vi "UltraScanning.vi"() -> ()   [LabVIEW 2014]
uses:
  <vilib>/userdefined/High Color/nirio_resource_hc.ctl
  <vilib>/Instr/_visa.llb/VISA Configure Serial Port (Instr).vi
  <vilib>/FPGAPlugInAG/PCIe-7851R/niLvFpga_Open_PCIe-7851R.vi
  <vilib>/rvi/interface/common/dynamic/niFpgaDynamicAddResources.vi
  <vilib>/Utility/error.llb/Error Cluster From Error Code.vi
  <vilib>/rvi/errors/niLvFpgaAdjustHostInterfaceError.vi
  <vilib>/FPGAPlugInAG/Dynamic/niLvFpga_Close_Dynamic.vi
  <vilib>/rvi/interface/nirviOpenFPGA/nirviOpenFPGA.xnode
  FPGA Bitfiles/FastHoppingModel_FPGATarget_StepApproach_dPgqUSt0PIw.lvbitx
  <vilib>/rvi/interface/nirviReadWriteControl/nirviReadWriteControl.xnode
  <vilib>/rvi/interface/nirviMethod/nirviMethod.xnode
  <vilib>/rvi/interface/nirviCloseFPGA/nirviCloseFPGA.xnode
  NiFpgaLv.dll
  <vilib>/rvi/interface/Simulation/niFpgaSimulationCallBeginRW.vi
  <vilib>/FPGAPlugInAG/Dynamic/niLvFpga_ReadFifo_Dynamic.vi
  <vilib>/rvi/errors/niLvFpgaMergeErrorWithErrorCode.vi
  CloseScanning.dll
  DeepScanning.dll
panel:
  out "Before":i16[][](array[numeric])
  out "After":u32[][](array[numeric])
  out "XNum?":i32
  out "YNum?":i32
  in  "SeveralSampleMeasure?":bool
  out "Intensity Graph":i32[][](graph)
  in  "Precise Scan Stop":bool
  out "RoughZPos um":dbl
  in  "steepWithdrawZIndex":i32
  in  "WithdrawZIndex":i32
  out "TimeDelta":u32
  in  "Prescan Stop":bool
  in  "PIZ":T1
  out "YPos um":dbl format="%#_13g"
  out "XPos um":dbl
  in  "InitOffset":i32
  in  "ApproachRate us":i32
  in  "Threshold %":dbl
  in  "YNum":i32
  in  "XNum":i32
  in  "XInitPos um":dbl
  in  "YInitPos um":dbl
  in  "YStepLen um":dbl
  in  "XStepLen um":dbl
  out "ERRIn?":string
  in  "RoughXYZ":refnum<visa-resource-name>
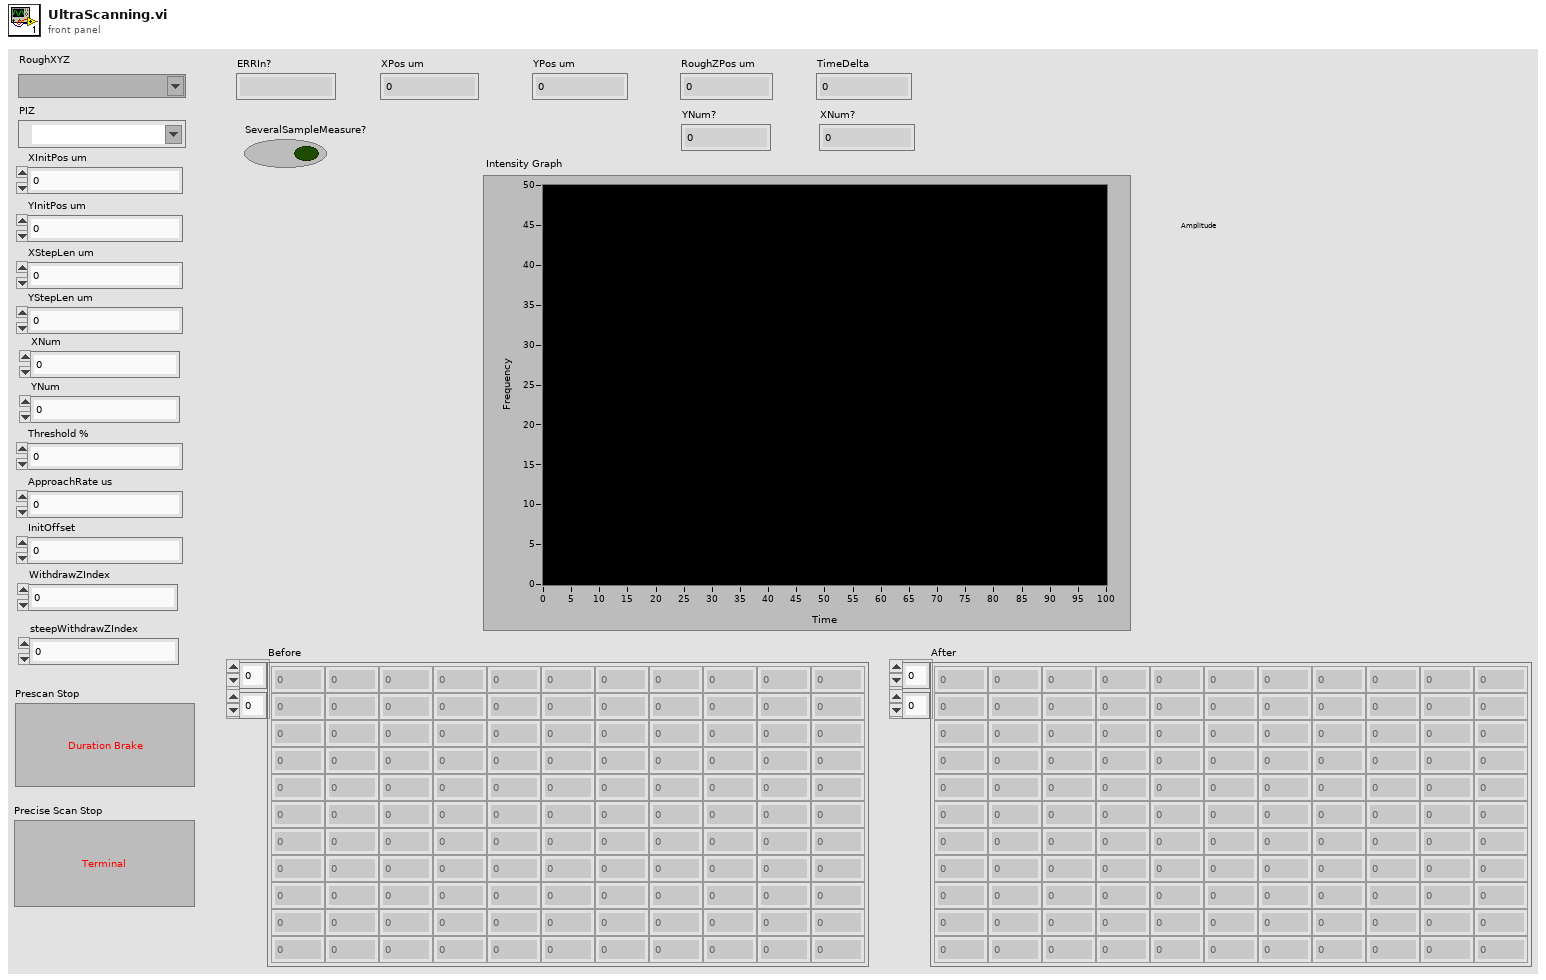
[diagram p1: front panel]
types:
  T1 = typedef "nirio_resource_hc.ctl" = tag
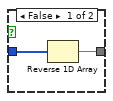
[diagram p2: hidden frame]
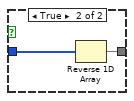
[diagram p5: hidden frame]
diagram:
  n1 = flat-sequence {
    tunnel: [w120] -> w98
    tunnel: [w119] -> w97
    tunnel: w98 -> [w148]
    tunnel: w97 -> [w147]
    tunnel: [w130] -> w96
    tunnel: [w129] -> w95
    tunnel: w96 -> [w150]
    tunnel: w95 -> [w149]
    tunnel: [w150] -> w94
    tunnel: [w149] -> w93
    tunnel: w94 -> [w177]
    tunnel: w93 -> [w176]
    tunnel: [w156] -> w92
    tunnel: [w155] -> w91
    tunnel: w92 -> [w179]
    tunnel: w91 -> [w178]
    tunnel: [w179] -> w90
    tunnel: [w178] -> w89
    tunnel: w90 -> [w189]
    tunnel: w89 -> [w188]
    tunnel: [w186] -> w88
    tunnel: [w185] -> w87
    tunnel: [w184] -> w86
    tunnel: [w183] -> w85
    tunnel: [w182] -> w84
    tunnel: [w181] -> w42
    tunnel: w88 -> [w401]
    tunnel: w87 -> [w403]
    tunnel: w86 -> [w402]
    tunnel: w85 -> [w399]
    tunnel: w84 -> [w398]
    tunnel: [w399] -> w49
    tunnel: [w398] -> w47
    tunnel: [w401] -> w45
    tunnel: [w400] -> w43
    tunnel: w42 -> [w400]
    tunnel: [w399] -> w41
    tunnel: [w398] -> w40
    tunnel: w49 -> [w410]
    tunnel: [w408] -> w48
    tunnel: w47 -> [w409]
    tunnel: [w407] -> w46
    tunnel: w45 -> [w412]
    tunnel: [w412] -> w44
    tunnel: w43 -> [w411]
    tunnel: w41 -> [w408]
    tunnel: w40 -> [w407]
    tunnel: w48 -> [w449]
    tunnel: w46 -> [w448]
    tunnel: w44 -> [w447]
    tunnel: [w449] -> w81
    tunnel: [w448] -> w79
    tunnel: [w436] -> w77
    tunnel: [w434] -> w74
    tunnel: [w438] -> w73
    tunnel: [w437] -> w72
    tunnel: [w439] -> w66
    tunnel: [w443] -> w64
    tunnel: [w442] -> w62
    tunnel: [w432] -> w60
    tunnel: [w435] -> w8
    tunnel: [w433] -> w7
    tunnel: [w431] -> w1
    tunnel: w81 -> [w465]
    tunnel: [w465] -> w80
    tunnel: w79 -> [w464]
    tunnel: [w464] -> w78
    tunnel: w77 -> [w463]
    tunnel: [w463] -> w76
    tunnel: [w462] -> w75
    tunnel: w74 -> [w457]
    tunnel: w73 -> [w459]
    tunnel: w72 -> [w458]
    tunnel: [w459] -> w71
    tunnel: [w458] -> w70
    tunnel: [w457] -> w69
    tunnel: [w456] -> w68
    tunnel: [w455] -> w67
    tunnel: w66 -> [w455]
    tunnel: [w454] -> w65
    tunnel: w64 -> [w453]
    tunnel: [w453] -> w63
    tunnel: w62 -> [w452]
    tunnel: [w452] -> w61
    tunnel: w60 -> [w451]
    tunnel: [w451] -> w59
    tunnel: [w450] -> w57
    tunnel: w8 -> [w462]
    tunnel: w7 -> [w456]
    tunnel: w1 -> [w450]
    tunnel: w80 -> [w486]
    tunnel: w78 -> [w485]
    tunnel: w76 -> [w476]
    tunnel: w75 -> [w475]
    tunnel: [w486] -> w83
    tunnel: [w485] -> w82
    tunnel: w71 -> [w481]
    tunnel: w70 -> [w480]
    tunnel: w69 -> [w474]
    tunnel: w68 -> [w473]
    tunnel: w67 -> [w482]
    tunnel: w65 -> [w477]
    tunnel: w63 -> [w479]
    tunnel: w61 -> [w478]
    tunnel: w59 -> [w484]
    tunnel: [w484] -> w58
    tunnel: w57 -> [w483]
    tunnel: [w483] -> w56
    tunnel: [w469] -> w6
    tunnel: [w467] -> w5
    tunnel: [w466] -> w4
    tunnel: [w470] -> w3
    tunnel: [w468] -> w2
    tunnel: w83 -> [w504]
    tunnel: w82 -> [w503]
    tunnel: w58 -> [w492]
    tunnel: w56 -> [w491]
    tunnel: [w501] -> w55
    tunnel: [w500] -> w54
    tunnel: [w493] -> w38
    tunnel: [w492] -> w36
    tunnel: [w491] -> w33
    tunnel: [w490] -> w30
    tunnel: [w489] -> w27
    tunnel: [w488] -> w26
    tunnel: [w487] -> w21
    tunnel: w6 -> [w493]
    tunnel: w5 -> [w489]
    tunnel: w4 -> [w488]
    tunnel: w3 -> [w487]
    tunnel: w2 -> [w490]
    tunnel: w55 -> [w513]
    tunnel: w54 -> [w512]
    tunnel: [w513] -> w53
    tunnel: [w512] -> w52
    tunnel: [w511] -> w39
    tunnel: w38 -> [w511]
    tunnel: w36 -> [w510]
    tunnel: [w510] -> w34
    tunnel: w33 -> [w509]
    tunnel: [w509] -> w32
    tunnel: w30 -> [w508]
    tunnel: [w508] -> w29
    tunnel: w27 -> [w507]
    tunnel: w26 -> [w506]
    tunnel: [w507] -> w25
    tunnel: [w506] -> w23
    tunnel: w21 -> [w505]
    tunnel: [w505] -> w20
    tunnel: w53 -> [w548]
    tunnel: w52 -> [w547]
    tunnel: [w525] -> w51
    tunnel: [w524] -> w50
    tunnel: w39 -> [w521]
    tunnel: [w521] -> w37
    tunnel: [w520] -> w35
    tunnel: w34 -> [w520]
    tunnel: w32 -> [w519]
    tunnel: [w519] -> w31
    tunnel: w29 -> [w518]
    tunnel: [w518] -> w28
    tunnel: w25 -> [w517]
    tunnel: [w517] -> w24
    tunnel: w23 -> [w516]
    tunnel: [w516] -> w22
    tunnel: w20 -> [w515]
    tunnel: [w515] -> w19
    tunnel: w51 -> [w561]
    tunnel: w50 -> [w560]
    tunnel: w37 -> [w562]
    tunnel: w35 -> [w556]
    tunnel: w31 -> [w555]
    tunnel: w28 -> [w559]
    tunnel: w24 -> [w557]
    tunnel: w22 -> [w558]
    tunnel: w19 -> [w553]
    tunnel: [w552] -> w18
    tunnel: [w551] -> w16
    tunnel: [w550] -> w14
    tunnel: [w549] -> w12
    tunnel: w18 -> [w810]
    tunnel: [w810] -> w17
    tunnel: w16 -> [w809]
    tunnel: [w809] -> w15
    tunnel: w14 -> [w808]
    tunnel: [w808] -> w13
    tunnel: w12 -> [w807]
    tunnel: [w807] -> w11
    tunnel: w17 -> [_]
    tunnel: w15 -> [_]
    tunnel: w13 -> [w815]
    tunnel: w11 -> [w814]
    tunnel: [w812] -> w10
    tunnel: [w811] -> w9
    tunnel: w10 -> [w824]
    tunnel: w9 -> [w823]
    frame #0 {
      w106 = 0 ("x")
      n2 = Wait (ms)(milliseconds to wait=u32 1000) -> ()  [unwired: 1 out]
      n3 = local write "XNum"("XNum") -> ()
      n4 = local write "InitOffset"("InitOffset") -> ()
      n5 = local write "YNum"("YNum") -> ()
      n6 = local write "Threshold %"("Threshold %") -> ()
      n7 = local write "XInitPos um"("XInitPos um") -> ()
      n8 = local write "XStepLen um"("XStepLen um") -> ()
      n9 = local write "YInitPos um"("YInitPos um") -> ()
      n10 = local write "YStepLen um"("YStepLen um") -> ()
      n11 = local write "ApproachRate us"("ApproachRate us") -> ()
      n12 = Equal?(x=w106, y="steepWithdrawZIndex") -> (x = y?=w100:bool)
      n13 = Equal?(x=w106, y="WithdrawZIndex") -> (x = y?=w105:bool)
      n14 = call-poly "VISA Configure Serial Port"("VISA resource name"="RoughXYZ", "baud rate (9600)"=u32 115200) -> ("VISA resource name out"=w126:refnum<visa-resource-name>, "error out"=w125:errorcluster)  [unwired: 12 in]
      n15 = Select(t=400 ("x"), s=w105, f="WithdrawZIndex") -> (s? t:f=w103:i32)
      n16 = Select(t=1000 ("x"), s=w100, f="steepWithdrawZIndex") -> (s? t:f=w102:i32)
      n17 = local write "steepWithdrawZIndex"(w102) -> ()
      n18 = local write "WithdrawZIndex"(w103) -> ()
      n19 = VISA Write(VISA resource name=w126, write buffer="ERR?\n", error in (no error)=w125) -> (VISA resource name out=w123:refnum<visa-resource-name>, error out=w122:errorcluster)  [unwired: 1 out]
      n20 = VISA Read(VISA resource name=w123, byte count=u32 128, error in (no error)=w122) -> (VISA resource name out=w120:refnum<visa-resource-name>, read buffer=→"ERRIn?":string, error out=w119:errorcluster)  [unwired: 1 out]
    }
    frame #1 {
      w140 = "\n" ("string")
      n21 = local read "YInitPos um"() -> (w135:dbl)
      n22 = local read "XInitPos um"() -> (w138:dbl)
      n23 = Wait (ms)(milliseconds to wait=u32 100) -> ()  [unwired: 1 out]
      n24 = Number To Fractional String(number=w135, precision (6)=i16 10) -> (F-format string=w134:string)  [unwired: 2 in]
      n25 = Number To Fractional String(number=w138, precision (6)=i16 10) -> (F-format string=w133:string)  [unwired: 2 in]
      n26 = Concatenate Strings("MOV B " ("string"), w134, w140) -> (w131:string)
      n27 = Concatenate Strings("MOV A " ("string"), w133, w140) -> (w132:string)
      n28 = Concatenate Strings(w132, w131) -> (w142:string)
      n29 = VISA Write(VISA resource name=w148, write buffer="ONL 1 1 2 1 3 1\nSVO A 1\nSVO B 1\nSVO C 1\nMOV C 0\n", error in (no error)=w147) -> (VISA resource name out=w144:refnum<visa-resource-name>, error out=w143:errorcluster)  [unwired: 1 out]
      n30 = VISA Write(VISA resource name=w144, write buffer=w142, error in (no error)=w143) -> (VISA resource name out=w130:refnum<visa-resource-name>, error out=w129:errorcluster)  [unwired: 1 out]
    }
    frame #2 {
      n31 = Wait (ms)(milliseconds to wait=u32 100) -> ()  [unwired: 1 out]
    }
    frame #3 {
      w153 = 2 ("offset")
      w157 = u32 128 ("byte count")
      n32 = VISA Write(VISA resource name=w177, write buffer="POS? A\n", error in (no error)=w176) -> (VISA resource name out=w174:refnum<visa-resource-name>, error out=w173:errorcluster)  [unwired: 1 out]
      n33 = VISA Read(VISA resource name=w174, byte count=w157, error in (no error)=w173) -> (VISA resource name out=w172:refnum<visa-resource-name>, read buffer=w170:string, error out=w171:errorcluster)  [unwired: 1 out]
      n34 = Fract/Exp String To Number(string=w170, offset=2) -> (number=→"XPos um":dbl)  [unwired: 2 in, 1 out]
      n35 = VISA Write(VISA resource name=w172, write buffer="POS? B\n", error in (no error)=w171) -> (VISA resource name out=w167:refnum<visa-resource-name>, error out=w166:errorcluster)  [unwired: 1 out]
      n36 = VISA Read(VISA resource name=w167, byte count=w157, error in (no error)=w166) -> (VISA resource name out=w162:refnum<visa-resource-name>, read buffer=w164:string, error out=w161:errorcluster)  [unwired: 1 out]
      n37 = Fract/Exp String To Number(string=w164, offset=w153) -> (number=→"YPos um":dbl)  [unwired: 2 in, 1 out]
      n38 = VISA Write(VISA resource name=w162, write buffer="POS? C\n", error in (no error)=w161) -> (VISA resource name out=w159:refnum<visa-resource-name>, error out=w158:errorcluster)  [unwired: 1 out]
      n39 = VISA Read(VISA resource name=w159, byte count=w157, error in (no error)=w158) -> (VISA resource name out=w156:refnum<visa-resource-name>, read buffer=w154:string, error out=w155:errorcluster)  [unwired: 1 out]
      n40 = Fract/Exp String To Number(string=w154, offset=w153) -> (number=→"RoughZPos um":dbl)  [unwired: 2 in, 1 out]
    }
    frame #4 {
      n41 = Wait (ms)(milliseconds to wait=u32 100) -> ()  [unwired: 1 out]
    }
    frame #5 {
      n42 = local read "YNum"() -> (w190:i32)
      n43 = for {
        N: w190 -> [_]
        tunnel: w189 -> [w224]
        tunnel: w188 -> [w223]
        shift-right: [w211] -> _
        shift-left: 0 -> [w217]
        tunnel: [w197] -> w183
        tunnel: [w196] -> w182
        tunnel: [w195] -> w185 mode=indexing
        tunnel: [w194] -> w184 mode=indexing
        tunnel: [w193] -> w186 mode=indexing
        tunnel: [w192] -> w181
        i -> [w191]
        stop <- w192 stop-if-true
        n44 = flat-sequence {
          tunnel: w191 -> [w249]
          tunnel: [w243] -> w225
          tunnel: w224 -> [w242]
          tunnel: w223 -> [w241]
          tunnel: [w240] -> w222
          tunnel: [w239] -> w221
          tunnel: w191 -> [w232]
          tunnel: [w228] -> w218
          tunnel: w217 -> [w228]
          tunnel: [w227] -> w206
          tunnel: w191 -> [w226]
          tunnel: w225 -> [w251]
          tunnel: w222 -> [w254]
          tunnel: w221 -> [w253]
          tunnel: [w254] -> w220
          tunnel: [w253] -> w219
          tunnel: w218 -> [w252]
          tunnel: [w252] -> w216
          tunnel: [w251] -> w215
          tunnel: [w250] -> w207
          tunnel: w206 -> [w250]
          tunnel: w220 -> [w268]
          tunnel: w219 -> [w267]
          tunnel: w216 -> [w265]
          tunnel: w215 -> [w266]
          tunnel: [w263] -> w214
          tunnel: [w262] -> w212
          tunnel: [w261] -> w209
          tunnel: w207 -> [w260]
          tunnel: [w260] -> w204
          tunnel: [w259] -> w202
          tunnel: [w258] -> w200
          tunnel: [w257] -> w198
          tunnel: w214 -> [w375]
          tunnel: [w375] -> w213
          tunnel: w212 -> [w374]
          tunnel: [w374] -> w210
          tunnel: w209 -> [w373]
          tunnel: [w373] -> w208
          tunnel: [w372] -> w205
          tunnel: w204 -> [w372]
          tunnel: [w371] -> w203
          tunnel: w202 -> [w371]
          tunnel: [w370] -> w201
          tunnel: w200 -> [w370]
          tunnel: [w368] -> w199
          tunnel: w198 -> [w368]
          tunnel: w213 -> [w393]
          tunnel: [w392] -> w211
          tunnel: w210 -> [w392]
          tunnel: [w391] -> w192
          tunnel: w208 -> [w391]
          tunnel: w205 -> [w390]
          tunnel: w203 -> [w383]
          tunnel: w201 -> [w382]
          tunnel: w199 -> [w389]
          tunnel: [w388] -> w193
          tunnel: [w381] -> w197
          tunnel: [w380] -> w196
          tunnel: [w379] -> w195
          tunnel: [w376] -> w194
          frame #0 {
            n45 = local read "YStepLen um"() -> (w233:dbl)
            n46 = local read "YInitPos um"() -> (w231:dbl)
            n47 = Multiply(x=w232, y=w233) -> (x*y=w230:dbl)
            n48 = Add(x=w231, y=w230) -> (x+y=w229:dbl)
            n49 = Number To Fractional String(number=w229, precision (6)=i16 10) -> (F-format string=w234:string)  [unwired: 2 in]
            n50 = Quotient & Remainder(x=w249, y=2) -> (x-y*floor(x/y)=w247:i32)  [unwired: 1 out]
            n51 = Concatenate Strings("MOV B " ("string"), w234, "\n" ("string")) -> (w238:string)
            n52 = Equal?(x=w247, y=0) -> (x = y?=w227:bool)
            n53 = VISA Write(VISA resource name=w242, write buffer=w238, error in (no error)=w241) -> (VISA resource name out=w240:refnum<visa-resource-name>, error out=w239:errorcluster)  [unwired: 1 out]
            n54 = Select(t=1, s=w227, f=-1) -> (s? t:f=w243:i32)
            "YNum?" <- w226
          }
          frame #1 {
            n55 = Wait (ms)(milliseconds to wait=u32 5) -> ()  [unwired: 1 out]
          }
          frame #2 {
            n56 = local read "XNum"() -> (w264:i32)
            n57 = Tick Count (ms)() -> (millisecond timer value=w256:u32)
            n58 = for {
              N: w264 -> [_]
              tunnel: w268 -> [w305]
              tunnel: w267 -> [w304]
              tunnel: w266 -> [w303]
              tunnel: w265 -> [w275]
              tunnel: [w278] -> w259
              tunnel: [w277] -> w258
              tunnel: [w276] -> w263 mode=indexing
              tunnel: [w274] -> w262
              tunnel: [w273] -> w261
              tunnel: [w271] -> w257 mode=indexing
              shift-right: [w269] -> _
              shift-left: w256 -> [w270]
              i -> [w302]
              stop <- w273 stop-if-true
              n59 = local read "XStepLen um"() -> (w300:dbl)
              n60 = Multiply(x=w302, y=w303) -> (x*y=w301:i32)
              n61 = local read "XInitPos um"() -> (w298:dbl)
              n62 = Add(x=w275, y=w301) -> (x+y=w274:i32)
              n63 = Multiply(x=w300, y=w274) -> (x*y=w299:dbl)
              n64 = Add(x=w298, y=w299) -> (x+y=w297:dbl)
              n65 = flat-sequence {
                tunnel: w305 -> [w315]
                tunnel: w304 -> [w314]
                tunnel: w297 -> [w309]
                tunnel: [w307] -> w296
                tunnel: [w306] -> w295
                tunnel: w296 -> [w317]
                tunnel: w295 -> [w316]
                tunnel: [w317] -> w294
                tunnel: [w316] -> w293
                tunnel: w294 -> [w326]
                tunnel: w293 -> [w325]
                tunnel: [w328] -> w292
                tunnel: [w327] -> w291
                tunnel: [w326] -> w290
                tunnel: [w325] -> w289
                tunnel: w292 -> [w343]
                tunnel: w291 -> [w342]
                tunnel: w290 -> [w336]
                tunnel: w289 -> [w335]
                tunnel: [w337] -> w288
                tunnel: [w336] -> w285
                tunnel: [w335] -> w283
                tunnel: [w334] -> w281
                tunnel: [w333] -> w279
                tunnel: ["Prescan Stop"] -> w273
                tunnel: w288 -> [w348]
                tunnel: [w348] -> w287
                tunnel: [w347] -> w286
                tunnel: w285 -> [w347]
                tunnel: [w346] -> w284
                tunnel: w283 -> [w346]
                tunnel: [w345] -> w282
                tunnel: w281 -> [w345]
                tunnel: [w344] -> w280
                tunnel: w279 -> [w344]
                tunnel: w287 -> [w356]
                tunnel: w286 -> [w365]
                tunnel: w284 -> [w364]
                tunnel: w282 -> [w367]
                tunnel: w280 -> [w366]
                tunnel: [w360] -> w278
                tunnel: [w359] -> w277
                tunnel: [w355] -> w271
                tunnel: [w352] -> w276
                tunnel: [w351] -> w269
                frame #0 {
                  n66 = Number To Fractional String(number=w309, precision (6)=i16 10) -> (F-format string=w308:string)  [unwired: 2 in]
                  n67 = Concatenate Strings("MOV B " ("string"), w308, "\n" ("string")) -> (w311:string)
                  n68 = VISA Write(VISA resource name=w315, write buffer=w311, error in (no error)=w314) -> (VISA resource name out=w307:refnum<visa-resource-name>, error out=w306:errorcluster)  [unwired: 1 out]
                }
                frame #1 {
                  n69 = Wait (ms)(milliseconds to wait=u32 5) -> ()  [unwired: 1 out]
                }
                frame #2 {
                  n70 = local read "ApproachRate us"() -> (w322:i32)
                  n71 = local read "Threshold %"() -> (w324:dbl)
                  n72 = local read "InitOffset"() -> (w323:i32)
                  n73 = xnode "Open FPGA VI Reference"("resource name"="PIZ") -> ("FPGA VI Reference Out"=w330:refnum<k20>, "error out"=w329:errorcluster)  [unwired: 1 in]
                  n74 = xnode "Read/Write Control"("FPGA VI Reference In"=w330, "error in"=w329, "Percentage %"=w324, "Offset"=w323, "AppRate us"=w322, "BaseTime us"=500, "CurrSampleNum"=100, "SeveralSampleMeasure?"="SeveralSampleMeasure?") -> ("FPGA VI Reference Out"=w328:refnum<k20>, "error out"=w327:errorcluster)
                }
                frame #3 {
                  n75 = xnode "Read/Write Control"("FPGA VI Reference In"=w343, "error in"=w342, "stop"="Prescan Stop") -> ("FPGA VI Reference Out"=w341:refnum<k20>, "error out"=w340:errorcluster)
                  n76 = xnode "Invoke Method"("FPGA VI Reference In"=w341, "error in"=w340, "Number of Elements"=u32 1, "Timeout (ms)"=7000) -> ("FPGA VI Reference Out"=w334:refnum<k20>, "error out"=w333:errorcluster, "Data"=w337:i16[])  [unwired: 1 out]
                }
                frame #4 {
                  n77 = Wait (ms)(milliseconds to wait=u32 1) -> ()  [unwired: 1 out]
                }
                frame #5 {
                  n78 = xnode "Close FPGA VI Reference"("FPGA VI Reference In"=w367, "error in"=w366) -> ()  [unwired: 1 out]
                  n79 = Array Size(array=w356) -> (size(s)=w358:i32)
                  n80 = VISA Write(VISA resource name=w365, write buffer="POS? A\n", error in (no error)=w364) -> (VISA resource name out=w362:refnum<visa-resource-name>, error out=w361:errorcluster)  [unwired: 1 out]
                  n81 = Decrement(x=w358) -> (x-1=w357:i32)
                  n82 = VISA Read(VISA resource name=w362, byte count=u32 128, error in (no error)=w361) -> (VISA resource name out=w360:refnum<visa-resource-name>, read buffer=w353:string, error out=w359:errorcluster)  [unwired: 1 out]
                  n83 = Index Array(array=w356, index=w357) -> (element=w355:i16)
                  n84 = Fract/Exp String To Number(string=w353, offset=2) -> (number=w352:dbl)  [unwired: 2 in, 1 out]
                  n85 = local write "XPos um"(w352) -> ()
                  n86 = Tick Count (ms)() -> (millisecond timer value=w351:u32)
                }
              }
              n87 = Subtract(x=w269, y=w270) -> (x-y=→"TimeDelta":u32)
              "XNum?" <- w302
            }
          }
          frame #3 {
            n88 = Wait (ms)(milliseconds to wait=u32 2) -> ()  [unwired: 1 out]
          }
          frame #4 {
            n89 = Index Array(array=w393, index=0) -> (element=w379:dbl)
            n90 = VISA Write(VISA resource name=w383, write buffer="POS? B\n", error in (no error)=w382) -> (VISA resource name out=w386:refnum<visa-resource-name>, error out=w385:errorcluster)  [unwired: 1 out]
            n91 = case shown="True" w390 {
              tunnel: w389 -> [w396 w397]
              tunnel: [w395 w397] -> w388
              frame False {
                n92 = Reverse 1D Array(array=w396) -> (reversed array=w395:i16[])
              }
              frame True {
              }
            }
            n93 = VISA Read(VISA resource name=w386, byte count=u32 128, error in (no error)=w385) -> (VISA resource name out=w381:refnum<visa-resource-name>, read buffer=w378:string, error out=w380:errorcluster)  [unwired: 1 out]
            n94 = Fract/Exp String To Number(string=w378, offset=2) -> (number=w376:dbl)  [unwired: 2 in, 1 out]
          }
        }
      }
    }
    frame #6 {
      n95 = call "Display Message to User"() -> ("OK"=w404:bool)  [unwired: 10 in, 1 out]
      n96 = case shown="True" w404 {
        tunnel: w401 -> [_ w406]
        tunnel: w403 -> [_ _]
        tunnel: w402 -> [_ _]
        frame False {
        }
        frame True {
          n97 = call "Convert to Dynamic Data"("2D Array"=w406) -> ("Dynamic Data Type"=w405:dynamicdata)  [unwired: 3 in]
          n98 = call "Write To Measurement File"("Signals"=w405) -> ()  [unwired: 16 in, 3 out]
        }
      }
    }
    frame #7 {
      n99 = case shown="True" w411 {
        selector: w411 -> [_ w415]
        tunnel: w410 -> [_ w417]
        tunnel: w409 -> [_ w416]
        frame False {
        }
        frame True {
          n100 = flat-sequence {
            tunnel: w417 -> [w427]
            tunnel: w416 -> [w426]
            tunnel: w415 -> [w425]
            tunnel: [w425] -> w414
            tunnel: w414 -> [w428]
            tunnel: [w428] -> w413
            tunnel: w413 -> [w430]
            frame #0 {
              n101 = VISA Write(VISA resource name=w427, write buffer="MOV A 0\nMOV B 0\nERR?\n", error in (no error)=w426) -> (VISA resource name out=w423:refnum<visa-resource-name>, error out=w422:errorcluster)  [unwired: 1 out]
              n102 = VISA Read(VISA resource name=w423, byte count=u32 128, error in (no error)=w422) -> (VISA resource name out=w419:refnum<visa-resource-name>, read buffer=w420:string, error out=w418:errorcluster)  [unwired: 1 out]
              n103 = VISA Close(VISA resource name=w419, error in (no error)=w418) -> ()  [unwired: 1 out]
              n104 = local write "ERRIn?"(w420) -> ()
            }
            frame #1 {
              n105 = Wait (ms)(milliseconds to wait=u32 100) -> ()  [unwired: 1 out]
            }
            frame #2 {
              n106 = Stop(stop? (T)=w430) -> ()
            }
          }
        }
      }
      "Before" <- w412
    }
    frame #8 {
      w444 = 0
      n107 = local read "YStepLen um"() -> (w442:dbl)
      n108 = local read "XStepLen um"() -> (w443:dbl)
      n109 = local read "XInitPos um"() -> (w441:dbl)
      n110 = local read "YInitPos um"() -> (w440:dbl)
      n111 = local read "XNum"() -> (w445:i32)
      n112 = local read "YNum"() -> (w446:i32)
      n113 = dll-call lib="F:/Programming/FastHopping/DeepScanning.dll" fn="?WinStart@@YAXPAK0000PAN111@Z"("dataArr"=w447, "arrRow"=w446, "arrCol"=w445, "preciseRow"=w444, "preciseCol"=w444, "XStepLen"=w443, "YStepLen"=w442, "XInitPos"=w441, "YInitPos"=w440) -> ("dataArr"=w439:u32[][], "arrRow"=w438:u32, "arrCol"=w437:u32, "preciseRow"=w436:u32, "preciseCol"=w435:u32, "XStepLen"=w434:dbl, "YStepLen"=w433:dbl, "XInitPos"=w432:dbl, "YInitPos"=w431:dbl)  [unwired: 4 in, 2 out]
    }
    frame #9 {
      n114 = Wait (ms)(milliseconds to wait=u32 50) -> ()  [unwired: 1 out]
      n115 = Initialize Array(i16 0, w459, w458) -> (w454:i16[][])
      "After" <- w455
    }
    frame #10 {
      n116 = local read "steepWithdrawZIndex"() -> (w471:i32)
      n117 = local read "WithdrawZIndex"() -> (w472:i32)
      n118 = dll-call lib="F:/Programming/FastHopping/CloseScanning.dll" fn="?closeScan@@YAXPAKKKNN0KKNNKK@Z"("originalArr"=w482, "originalRowNum"=w481, "originalColNum"=w480, "originalXStep"=w479, "originalYStep"=w478, "preciseArr"=w477, "preciseRowNum"=w476, "preciseColNum"=w475, "preciseXStep"=w474, "preciseYStep"=w473, "withdrawZIndex"=w472, "steepWithdrawZIndex"=w471) -> ("preciseArr"=w470:u32[][], "preciseRowNum"=w469:u32, "preciseColNum"=w468:u32, "preciseXStep"=w467:dbl, "preciseYStep"=w466:dbl)  [unwired: 11 in, 2 out]
    }
    frame #11 {
      w497 = i16 10 ("precision (6)")
      n119 = Number To Fractional String(number=w492, precision (6)=w497) -> (F-format string=w498:string)  [unwired: 2 in]
      n120 = Number To Fractional String(number=w491, precision (6)=w497) -> (F-format string=w496:string)  [unwired: 2 in]
      n121 = Concatenate Strings("MOV A " ("string"), w498, "\nMOV B " ("string"), w496, "\n" ("string")) -> (w502:string)
      n122 = VISA Write(VISA resource name=w504, write buffer=w502, error in (no error)=w503) -> (VISA resource name out=w501:refnum<visa-resource-name>, error out=w500:errorcluster)  [unwired: 1 out]
    }
    frame #12 {
      n123 = Wait (ms)(milliseconds to wait=u32 500) -> ()  [unwired: 1 out]
    }
    frame #13 {
      w526 = 2 ("offset")
      n124 = VISA Write(VISA resource name=w548, write buffer="POS? A\n", error in (no error)=w547) -> (VISA resource name out=w544:refnum<visa-resource-name>, error out=w545:errorcluster)  [unwired: 1 out]
      n125 = VISA Read(VISA resource name=w544, byte count=u32 128, error in (no error)=w545) -> (VISA resource name out=w536:refnum<visa-resource-name>, read buffer=w542:string, error out=w535:errorcluster)  [unwired: 1 out]
      n126 = Fract/Exp String To Number(string=w542, offset=w526) -> (number=w541:dbl)  [unwired: 2 in, 1 out]
      n127 = local write "XPos um"(w541) -> ()
      n128 = VISA Write(VISA resource name=w536, write buffer="POS? B\n", error in (no error)=w535) -> (VISA resource name out=w538:refnum<visa-resource-name>, error out=w539:errorcluster)  [unwired: 1 out]
      n129 = VISA Read(VISA resource name=w538, byte count=u32 128, error in (no error)=w539) -> (VISA resource name out=w528:refnum<visa-resource-name>, read buffer=w534:string, error out=w527:errorcluster)  [unwired: 1 out]
      n130 = Fract/Exp String To Number(string=w534, offset=w526) -> (number=w533:dbl)  [unwired: 2 in, 1 out]
      n131 = local write "YPos um"(w533) -> ()
      n132 = VISA Write(VISA resource name=w528, write buffer="POS? C\n", error in (no error)=w527) -> (VISA resource name out=w530:refnum<visa-resource-name>, error out=w531:errorcluster)  [unwired: 1 out]
      n133 = VISA Read(VISA resource name=w530, byte count=u32 128, error in (no error)=w531) -> (VISA resource name out=w525:refnum<visa-resource-name>, read buffer=w523:string, error out=w524:errorcluster)  [unwired: 1 out]
      n134 = Fract/Exp String To Number(string=w523, offset=w526) -> (number=w522:dbl)  [unwired: 2 in, 1 out]
      n135 = local write "RoughZPos um"(w522) -> ()
    }
    frame #14 {
      n136 = for {
        N: w562 -> [_]
        tunnel: w561 -> [w612]
        tunnel: w560 -> [w611]
        tunnel: w559 -> [w609]
        tunnel: w558 -> [w608]
        tunnel: w557 -> [w606]
        tunnel: w556 -> [w605]
        tunnel: w555 -> [w604]
        shift-right: [w587] -> _
        shift-left: 0 -> [w588]
        tunnel: w553 -> [w586]
        tunnel: [w568] -> w550
        tunnel: [w567] -> w549
        tunnel: [w564] -> w552 mode=indexing
        tunnel: [w563] -> w551 mode=indexing
        i -> [w610]
        stop <- w581 stop-if-true
        n137 = flat-sequence {
          tunnel: w612 -> [w638]
          tunnel: w611 -> [w637]
          tunnel: w610 -> [w613]
          tunnel: w609 -> [w625]
          tunnel: w608 -> [w634]
          tunnel: [w633] -> w607
          tunnel: w606 -> [w633]
          tunnel: w605 -> [w630]
          tunnel: w604 -> [w631]
          tunnel: [w630] -> w603
          tunnel: [w625] -> w601
          tunnel: [w624] -> w599
          tunnel: [w623] -> w597
          tunnel: [w617] -> w595
          tunnel: [w616] -> w593
          tunnel: [w615] -> w589
          tunnel: w588 -> [w615]
          tunnel: w586 -> [w614]
          tunnel: [w614] -> w584
          tunnel: [w613] -> w582
          tunnel: w607 -> [w643]
          tunnel: w603 -> [w642]
          tunnel: [w648] -> w602
          tunnel: w601 -> [w648]
          tunnel: [w647] -> w600
          tunnel: w599 -> [w647]
          tunnel: [w646] -> w598
          tunnel: w597 -> [w646]
          tunnel: [w645] -> w596
          tunnel: w595 -> [w645]
          tunnel: [w644] -> w594
          tunnel: w593 -> [w644]
          tunnel: [w643] -> w592
          tunnel: [w642] -> w591
          tunnel: [w641] -> w590
          tunnel: w589 -> [w641]
          tunnel: [w640] -> w585
          tunnel: w584 -> [w640]
          tunnel: [w639] -> w583
          tunnel: w582 -> [w639]
          tunnel: w602 -> [w667]
          tunnel: w600 -> [w664]
          tunnel: w598 -> [w663]
          tunnel: w596 -> [w655]
          tunnel: w594 -> [w665]
          tunnel: w592 -> [w662]
          tunnel: w591 -> [w661]
          tunnel: w590 -> [w660]
          tunnel: [w659] -> w580
          tunnel: w585 -> [w658]
          tunnel: w583 -> [w657]
          tunnel: [w656] -> w578
          tunnel: [w655] -> w576
          tunnel: [w654] -> w574
          tunnel: [w653] -> w571
          tunnel: [w652] -> w569
          tunnel: [w651] -> w565
          tunnel: w580 -> [w786]
          tunnel: [w786] -> w579
          tunnel: w578 -> [w785]
          tunnel: [w785] -> w577
          tunnel: w576 -> [w784]
          tunnel: [w784] -> w575
          tunnel: w574 -> [w783]
          tunnel: [w783] -> w573
          tunnel: [w781] -> w572
          tunnel: w571 -> [w781]
          tunnel: [w780] -> w570
          tunnel: w569 -> [w780]
          tunnel: [w779] -> w566
          tunnel: w565 -> [w779]
          tunnel: w579 -> [w802]
          tunnel: [w802] -> w587
          tunnel: w577 -> [w801]
          tunnel: [w801] -> w581
          tunnel: w575 -> [w790]
          tunnel: w573 -> [_]
          tunnel: w572 -> [w796]
          tunnel: w570 -> [w795]
          tunnel: [w794] -> w568
          tunnel: [w793] -> w567
          tunnel: w566 -> [w789]
          tunnel: [w788] -> w564
          tunnel: [w787] -> w563
          frame #0 {
            n138 = Multiply(x=w634, y=w613) -> (x*y=w632:dbl)
            n139 = Add(x=w631, y=w632) -> (x+y=w629:dbl)
            n140 = Number To Fractional String(number=w629, precision (6)=i16 10) -> (F-format string=w627:string)  [unwired: 2 in]
            n141 = Quotient & Remainder(x=w613, y=2) -> (x-y*floor(x/y)=w621:i32)  [unwired: 1 out]
            n142 = Concatenate Strings("MOV B " ("string"), w627, "\n" ("string")) -> (w636:string)
            n143 = Equal?(x=0, y=w621) -> (x = y?=w617:bool)
            n144 = VISA Write(VISA resource name=w638, write buffer=w636, error in (no error)=w637) -> (VISA resource name out=w624:refnum<visa-resource-name>, error out=w623:errorcluster)  [unwired: 1 out]
            n145 = Select(t=1, s=w617, f=-1) -> (s? t:f=w616:i32)
          }
          frame #1 {
            n146 = Wait (ms)(milliseconds to wait=u32 5) -> ()  [unwired: 1 out]
          }
          frame #2 {
            w650 = i32[] []
            n147 = Tick Count (ms)() -> (millisecond timer value=w666:u32)
            n148 = for {
              N: w667 -> [_]
              tunnel: w665 -> [w711]
              tunnel: w664 -> [w713]
              tunnel: w663 -> [w712]
              tunnel: w662 -> [w710]
              tunnel: w661 -> [w709]
              tunnel: w660 -> [w699]
              tunnel: [w699] -> w659
              tunnel: w658 -> [w697]
              tunnel: w657 -> [w694]
              tunnel: [w691] -> w656
              tunnel: [w690] -> w654 mode=indexing
              tunnel: [w682] -> w653
              tunnel: [w681] -> w652
              tunnel: [w679] -> w651 mode=indexing
              shift-right: [w676] -> _
              shift-left: w650 -> [w678]
              shift-right: [w675] -> _
              shift-left: w650 -> [w677]
              shift-right: [w673] -> _
              shift-left: w666 -> [w672]
              i -> [w680]
              stop <- w691 stop-if-true
              n149 = Multiply(x=w711, y=w680) -> (x*y=w700:i32)
              n150 = Add(x=w699, y=w700) -> (x+y=w698:i32)
              n151 = Multiply(x=w710, y=w698) -> (x*y=w708:dbl)
              n152 = Add(x=w709, y=w708) -> (x+y=w707:dbl)
              n153 = flat-sequence {
                tunnel: w713 -> [w724]
                tunnel: w712 -> [w723]
                tunnel: w707 -> [w719]
                tunnel: [w716] -> w706
                tunnel: [w715] -> w705
                tunnel: w697 -> [w714]
                tunnel: [w714] -> w695
                tunnel: w706 -> [w727]
                tunnel: w705 -> [w726]
                tunnel: [w727] -> w704
                tunnel: [w726] -> w703
                tunnel: [w725] -> w696
                tunnel: w695 -> [w725]
                tunnel: w704 -> [w730]
                tunnel: w703 -> [w729]
                tunnel: [w740] -> w702
                tunnel: [w739] -> w701
                tunnel: w698 -> [w737]
                tunnel: w696 -> [w738]
                tunnel: w694 -> [w736]
                tunnel: [w730] -> w693
                tunnel: [w729] -> w692
                tunnel: w702 -> [w755]
                tunnel: w701 -> [w754]
                tunnel: w693 -> [w752]
                tunnel: w692 -> [w751]
                tunnel: ["Precise Scan Stop"] -> w691
                tunnel: [w752] -> w688
                tunnel: [w751] -> w686
                tunnel: [w746] -> w684
                tunnel: [w745] -> w670
                tunnel: [w744] -> w669
                tunnel: w688 -> [w761]
                tunnel: [w761] -> w687
                tunnel: w686 -> [w760]
                tunnel: [w760] -> w685
                tunnel: w684 -> [w759]
                tunnel: [w759] -> w683
                tunnel: [w757] -> w671
                tunnel: w670 -> [w757]
                tunnel: w669 -> [w756]
                tunnel: [w756] -> w668
                tunnel: w687 -> [w772]
                tunnel: w685 -> [w771]
                tunnel: w683 -> [w778]
                tunnel: [w776] -> w679
                tunnel: [w770] -> w682
                tunnel: [w769] -> w681
                tunnel: [w767] -> w673
                tunnel: [w764] -> w690
                tunnel: w671 -> [w763]
                tunnel: w668 -> [w762]
                frame #0 {
                  n154 = Number To Fractional String(number=w719, precision (6)=i16 10) -> (F-format string=w718:string)  [unwired: 2 in]
                  n155 = Concatenate Strings("MOV B " ("string"), w718, "\n" ("string")) -> (w720:string)
                  n156 = VISA Write(VISA resource name=w724, write buffer=w720, error in (no error)=w723) -> (VISA resource name out=w716:refnum<visa-resource-name>, error out=w715:errorcluster)  [unwired: 1 out]
                }
                frame #1 {
                  n157 = Wait (ms)(milliseconds to wait=u32 5) -> ()  [unwired: 1 out]
                }
                frame #2 {
                  n158 = Index Array(array=w738, index (row)=w736, index (col)=w737) -> (element=w733:u32)
                  n159 = local read "PIZ"() -> (w743:T1)
                  n160 = local read "ApproachRate us"() -> (w734:i32)
                  n161 = local read "Threshold %"() -> (w735:dbl)
                  n162 = xnode "Open FPGA VI Reference"("resource name"=w743) -> ("FPGA VI Reference Out"=w742:refnum<k20>, "error out"=w741:errorcluster)  [unwired: 1 in]
                  n163 = xnode "Read/Write Control"("FPGA VI Reference In"=w742, "error in"=w741, "Percentage %"=w735, "Offset"=w733, "AppRate us"=w734, "BaseTime us"=500, "CurrSampleNum"=100) -> ("FPGA VI Reference Out"=w740:refnum<k20>, "error out"=w739:errorcluster)
                }
                frame #3 {
                  n164 = xnode "Read/Write Control"("FPGA VI Reference In"=w755, "error in"=w754, "stop"="Precise Scan Stop") -> ("FPGA VI Reference Out"=w750:refnum<k20>, "error out"=w749:errorcluster)
                  n165 = xnode "Invoke Method"("FPGA VI Reference In"=w750, "error in"=w749, "Number of Elements"=u32 1, "Timeout (ms)"=8000) -> ("FPGA VI Reference Out"=w745:refnum<k20>, "error out"=w744:errorcluster, "Data"=w746:i16[])  [unwired: 1 out]
                }
                frame #4 {
                  n166 = Wait (ms)(milliseconds to wait=u32 1) -> ()  [unwired: 1 out]
                }
                frame #5 {
                  n167 = xnode "Close FPGA VI Reference"("FPGA VI Reference In"=w763, "error in"=w762) -> ()  [unwired: 1 out]
                  n168 = VISA Write(VISA resource name=w772, write buffer="POS? A\n", error in (no error)=w771) -> (VISA resource name out=w774:refnum<visa-resource-name>, error out=w773:errorcluster)  [unwired: 1 out]
                  n169 = Index Array(array=w778, index=0) -> (element=w776:i16)
                  n170 = VISA Read(VISA resource name=w774, byte count=u32 128, error in (no error)=w773) -> (VISA resource name out=w770:refnum<visa-resource-name>, read buffer=w765:string, error out=w769:errorcluster)  [unwired: 1 out]
                  n171 = Fract/Exp String To Number(string=w765, offset=2) -> (number=w764:dbl)  [unwired: 2 in, 1 out]
                  n172 = local write "XPos um"(w764) -> ()
                  n173 = Tick Count (ms)() -> (millisecond timer value=w767:u32)
                }
              }
              n174 = Subtract(x=w673, y=w672) -> (x-y=w689:u32)
              n175 = Build Array (concatenate)(w680, w678) -> (w676:i32[])
              n176 = Build Array (concatenate)(w679, w677) -> (w675:i32[])
              n177 = local write "TimeDelta"(w689) -> ()
              n178 = Build Array(w676, w675) -> (→"Intensity Graph":i32[][])
            }
          }
          frame #3 {
            n179 = Wait (ms)(milliseconds to wait=u32 2) -> ()  [unwired: 1 out]
          }
          frame #4 {
            n180 = VISA Write(VISA resource name=w796, write buffer="POS? B\n", error in (no error)=w795) -> (VISA resource name out=w799:refnum<visa-resource-name>, error out=w798:errorcluster)  [unwired: 1 out]
            n181 = VISA Read(VISA resource name=w799, byte count=u32 128, error in (no error)=w798) -> (VISA resource name out=w794:refnum<visa-resource-name>, read buffer=w791:string, error out=w793:errorcluster)  [unwired: 1 out]
            n182 = case shown="False" w790 {
              tunnel: w789 -> [w803 w805]
              tunnel: [w803 w804] -> w788
              frame False {
              }
              frame True {
                n183 = Reverse 1D Array(array=w805) -> (reversed array=w804:i16[])
              }
            }
            n184 = Fract/Exp String To Number(string=w791, offset=2) -> (number=w787:dbl)  [unwired: 2 in, 1 out]
            n185 = local write "YPos um"(w787) -> ()
          }
        }
      }
    }
    frame #15 {
      n186 = Wait (ms)(milliseconds to wait=u32 100) -> ()  [unwired: 1 out]
    }
    frame #16 {
      n187 = VISA Write(VISA resource name=w815, write buffer="MOV A 0\nMOV B 0\n", error in (no error)=w814) -> (VISA resource name out=w812:refnum<visa-resource-name>, error out=w811:errorcluster)  [unwired: 1 out]
    }
    frame #17 {
      n188 = VISA Write(VISA resource name=w824, write buffer="ERR?\n", error in (no error)=w823) -> (VISA resource name out=w821:refnum<visa-resource-name>, error out=w820:errorcluster)  [unwired: 1 out]
      n189 = VISA Read(VISA resource name=w821, byte count=u32 128, error in (no error)=w820) -> (VISA resource name out=w817:refnum<visa-resource-name>, read buffer=w818:string, error out=w816:errorcluster)  [unwired: 1 out]
      n190 = VISA Close(VISA resource name=w817, error in (no error)=w816) -> ()  [unwired: 1 out]
      n191 = local write "ERRIn?"(w818) -> ()
    }
  }
